vi "_CSMOFGV Dequeue.vi"(8 "Error in":errorcluster caption="Error in (no error)", 9 "Dequeue Timeout(0ms)":i32, 10 "State(s) in (\"\")":string, 11 "CSMQ in":T1={"Requested Name"="", "Module Name"="", "Mode"=enum."Stand Alone", "Queue"=refnum, "CSM-Data"=refnum, "User Event"=refnum, "Status Change Event"=refnum, "Allowed Messages"=[], "Mode-Data"=refnum, "Group Name"="", "Exit Event"=refnum}) -> (0 "Error out":errorcluster, 2 "States Out":string, 3 "CSMQ out":T1={"Requested Name"="", "Module Name"="", "Mode"=enum."Stand Alone", "Queue"=refnum, "CSM-Data"=refnum, "User Event"=refnum, "Status Change Event"=refnum, "Allowed Messages"=[], "Mode-Data"=refnum, "Group Name"="", "Exit Event"=refnum})   [LabVIEW 2020, in "Communicable State Machine.lvlib"]
uses:
  Communicable State Machine.lvlib
  _CSMObj.ctl
  Priority Queue.lvclass
  _CSM_MODE.ctl
  _CSMObj-Data.ctl
  _CSM Status Change Event Data.ctl
  _CSMObj-ModeData.ctl
  Priority Queue.lvclass/Priority Queue.ctl
  CSM - Convert Error to Argument.vi
  CSM - Make String Arguments Safe.vi
  CSM - Keywords.vi
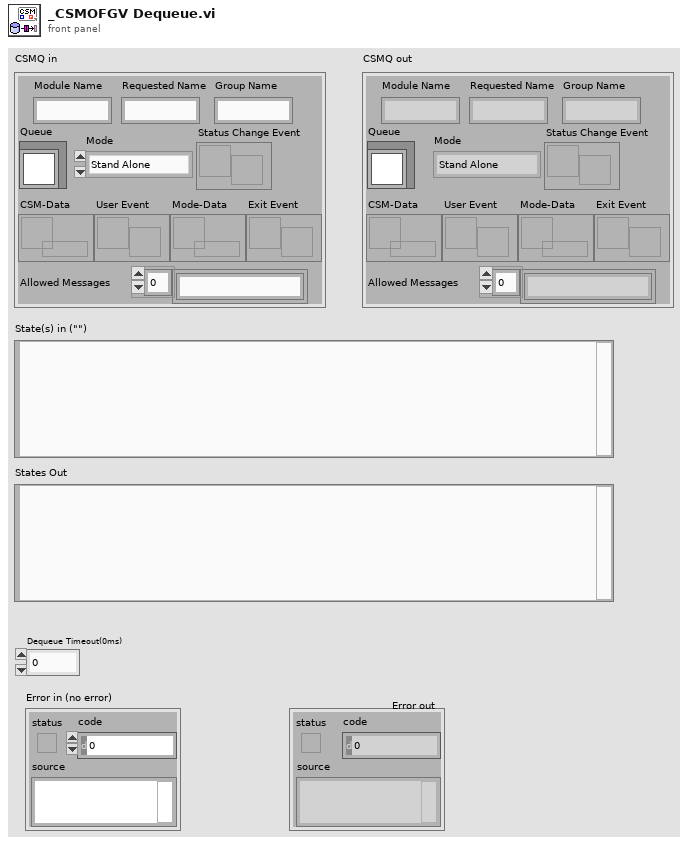
[diagram p1: front panel]
types:
  T1 = typedef "Communicable State Machine.lvlib/_CSMObj.ctl" = cluster{"Requested Name":string, "Module Name":string, "Mode":T2, "Queue":refnum<class "Priority Queue.lvclass">, "CSM-Data":refnum<data-value>, "User Event":refnum<user-event>, "Status Change Event":refnum<user-event>, "Allowed Messages":string[], "Mode-Data":refnum<data-value>, "Group Name":string, "Exit Event":refnum<user-event>}
  T2 = typedef "Communicable State Machine.lvlib/_CSM_MODE.ctl" = enum16{"Not Exist", "Stand Alone", "CSM", "Worker Agent", "Worker", "Chain", "Chain Node"}
  T3 = typedef "Communicable State Machine.lvlib/_CSMObj-Data.ctl" = cluster{"RemoteMessge?":bool, "error":errorcluster}
  T4 = typedef "Communicable State Machine.lvlib/_Cross CSM State Data.ctl" = cluster{"Msg Type":T5, "state":string, "args":string, "source":string, "RespQ":refnum<queue>, "Response For Message":T6, "Target":string}
  T5 = typedef "Communicable State Machine.lvlib/_CSM_MSG_TYPE.ctl" = enum16{"Sync Message(-@)", "Async Message(->)", "Async without Response(->|)", "Async Response", "Broadcast(-><all>)", "Broadcast(-><status>)", "Broadcast(-><interrupt>)", "Append to JKISM States", "Append to JKISM States(High Priority)"}
  T6 = typedef "Communicable State Machine.lvlib/_CSM_Response Source Message.ctl" = cluster{"‘State":string, "’Arguments":string, "’Error":errorcluster}
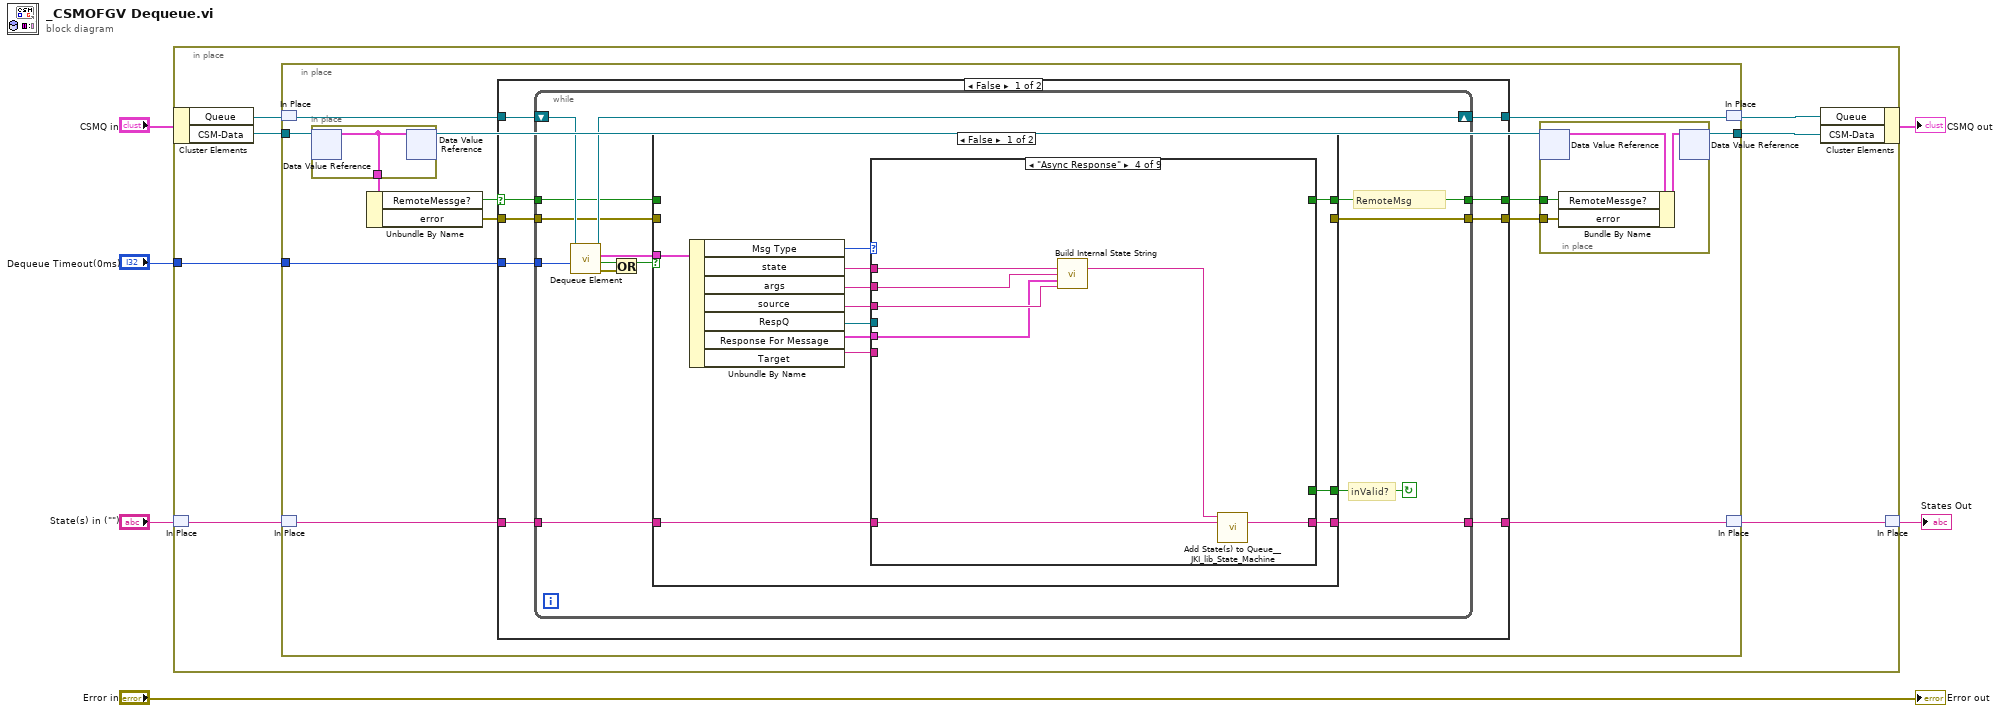
[diagram p0: block diagram]
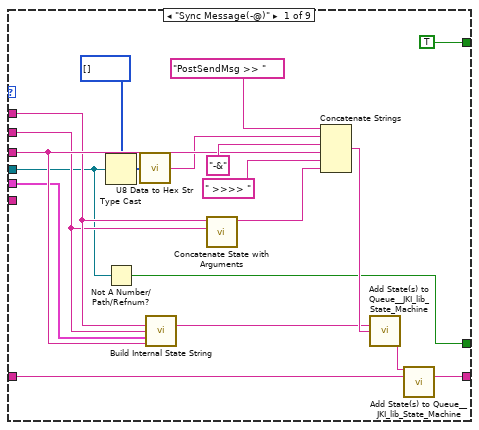
[diagram p2: hidden frame]
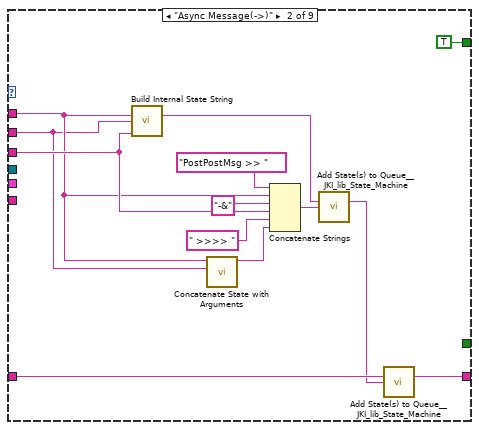
[diagram p3: hidden frame]
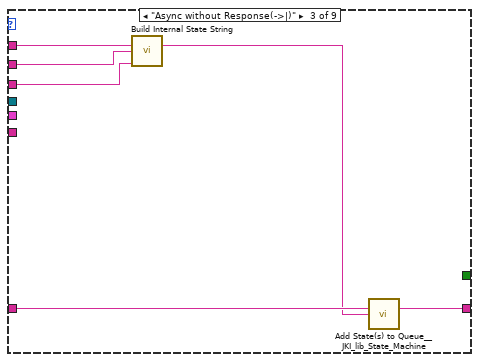
[diagram p4: hidden frame]
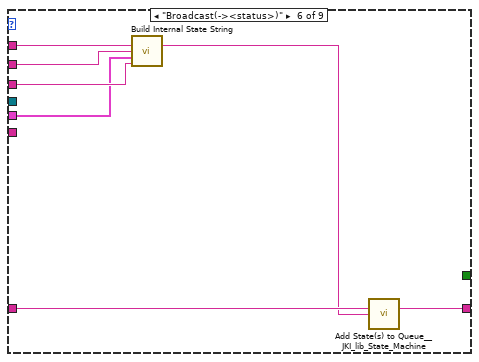
[diagram p6: hidden frame]
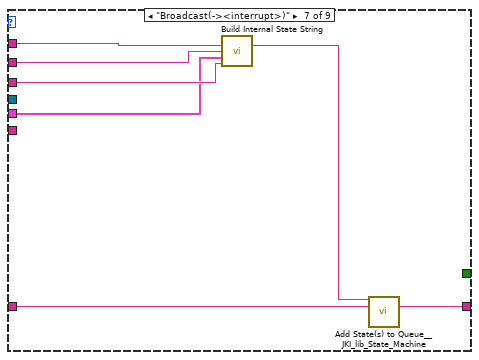
[diagram p7: hidden frame]
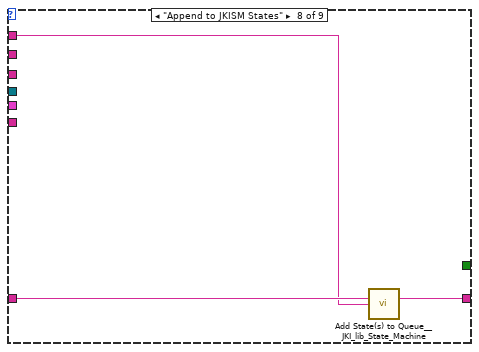
[diagram p8: hidden frame]
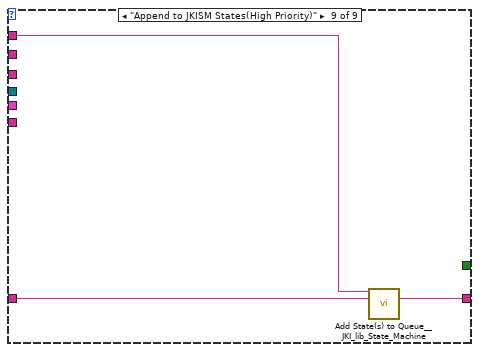
[diagram p9: hidden frame]
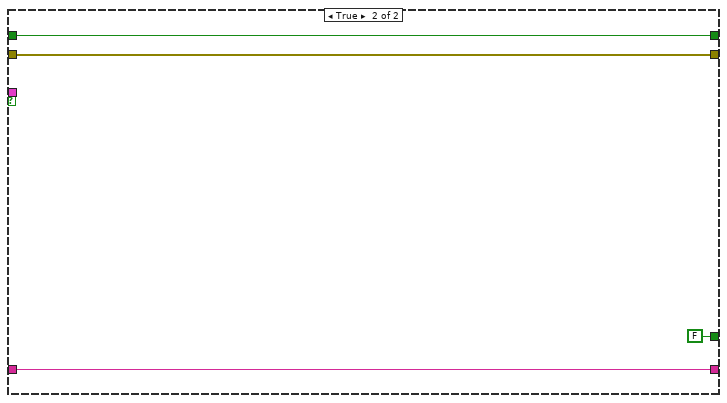
[diagram p10: hidden frame]
diagram:
  n1 = in-place "In Place Element Structure" {
    in-place-border: "Dequeue Timeout(0ms)" -> [w11]
    n2 = in-place-cluster #1("CSMQ in") -> ("Queue"=w13:refnum<class "Priority Queue.lvclass">, "CSM-Data"=w8:refnum<data-value>)
    n3 = in-place-match #2("State(s) in (\"\")") -> (w10:string)
    n4 = in-place {
      in-place-border: w11 -> [w24]
      in-place-border: w8 -> [w21]
      in-place-border: [w18] -> w7
      n5 = in-place-match #3(w13) -> (w25:refnum<class "Priority Queue.lvclass">)
      n6 = in-place-match #4(w10) -> (w23:string)
      n7 = in-place {
        in-place-border: [w31] -> w20
        n8 = in-place-dvr #5(w21) -> (w31:T3)  [unwired: 1 out]
        n9 = in-place-dvr #5(w31) -> (w19:refnum<data-value>)  [unwired: 1 out]
      }
      n10 = Unbundle By Name(w20) -> ("RemoteMessge?"=w16:bool, "error"=w14:errorcluster)
      n11 = case shown="False" w16 {
        selector: w16 -> [w34 w138]
        tunnel: [w39 w140] -> w26
        tunnel: w25 -> [w40 w140]
        tunnel: w24 -> [w38 _]
        tunnel: w23 -> [w37 w139]
        tunnel: [w36 w139] -> w22
        tunnel: [w35 w138] -> w17
        tunnel: [w33 w137] -> w15
        tunnel: w14 -> [w32 w137]
        frame False {
          n12 = while {
            tunnel: w38 -> [w52]
            shift-right: [w53] -> w39
            shift-left: w40 -> [w54]
            tunnel: w34 -> [w44]
            tunnel: [w45] -> w35
            tunnel: w37 -> [w50]
            tunnel: [w49] -> w36
            tunnel: [w42] -> w33
            tunnel: w32 -> [w41]
            stop <- w43 continue-if-true
            # "inValid?"
            # "RemoteMsg"
            n13 = call "Dequeue Element.vi"("timeout in ms (-1)"=w52, "Priority Queue"=w54) -> ("error out"=w46:errorcluster, "timed out?"=w47:bool, "Cross JKI State Machine State"=w51:T4, "Priority Queue(dup)"=w53:refnum<class "Priority Queue.lvclass">)  [unwired: 5 in, 1 out]
            n14 = Or(x=w47, y=w46) -> (x .or. y?=w48:bool)
            n15 = case shown="False" w48 {
              tunnel: w50 -> [w66 w136]
              tunnel: [w65 w136] -> w49
              tunnel: w51 -> [w60 _]
              tunnel: [w56 w135] -> w45
              tunnel: w44 -> [_ w135]
              tunnel: [w55 FALSE] -> w43
              tunnel: [_ w133] -> w42
              tunnel: w41 -> [_ w133]
              frame False {
                n16 = Unbundle By Name(w60) -> ("Msg Type"=w58:T5, "state"=w63:string, "args"=w62:string, "source"=w61:string, "RespQ"=w64:refnum<queue>, "Response For Message"=w59:T6, "Target"=w57:string)
                n17 = case shown="\"Async Response\"" w58 {
                  tunnel: w66 -> [w85 w98 w104 w111 w112 w119 w126 w129 w132]
                  tunnel: [w84 w97 w103 w110 w112 w118 w125 w128 w131] -> w65
                  tunnel: w64 -> [w68 _ _ _ _ _ _ _ _]
                  tunnel: w63 -> [w74 w87 w100 w107 _ w115 w122 w127 w130]
                  tunnel: w62 -> [w73 w86 w102 w109 _ w117 w124 _ _]
                  tunnel: w61 -> [w77 w96 w101 w108 _ w116 w123 _ _]
                  tunnel: w59 -> [w75 _ _ w105 _ w114 w121 _ _]
                  tunnel: w57 -> [_ _ _ _ _ _ _ _ _]
                  tunnel: [TRUE TRUE _ _ _ _ _ _ _] -> w56
                  tunnel: [w67 _ _ _ _ _ _ _ _] -> w55
                  frame "Sync Message(-@)" {
                    n18 = Type Cast(type=u8[] [], x=w68) -> (*(type *) &x=w70:u8[])
                    n19 = Not A Number/Path/Refnum?(number/path/refnum=w68) -> (NaN/Path/Refnum?=w67:bool)
                    n20 = call "U8 Data to Hex Str.vi"("u8 Data[]"=w70) -> ("HEX String (0-9,A-F)"=w69:string)
                    n21 = call "Build Internal State String.vi"("State"=w74, "Arguments (\"\")"=w73, ">> Response Source Message >>"=w75, "Source (\"\")"=w77) -> ("State with Arguments"=w80:string)  [unwired: 11 in]
                    n22 = call "Concatenate State with Arguments.vi"("Arguments"=w73, "State"=w74) -> ("State with Arguements"=w72:string)  [unwired: 9 in]
                    n23 = Concatenate Strings("PostSendMsg >> " ("State(s) at Back (\"\")"), w69, "-&" ("string"), w77, " >>>> " ("string"), w72) -> (w81:string)
                    n24 = call "Add State(s) to Queue__JKI_lib_State_Machine.vi"("State(s) in (\"\")"=w80, "State(s) at Back (\"\")"=w81) -> ("States Out"=w83:string)  [unwired: 13 in]
                    n25 = call "Add State(s) to Queue__JKI_lib_State_Machine.vi"("State(s) in Front (\"\")"=w83, "State(s) in (\"\")"=w85) -> ("States Out"=w84:string)  [unwired: 13 in]
                  }
                  frame "Async Message(->)" {
                    n26 = call "Build Internal State String.vi"("State"=w87, "Arguments (\"\")"=w86, "Source (\"\")"=w96) -> ("State with Arguments"=w92:string)  [unwired: 12 in]
                    n27 = call "Concatenate State with Arguments.vi"("Arguments"=w86, "State"=w87) -> ("State with Arguements"=w88:string)  [unwired: 9 in]
                    n28 = Concatenate Strings("PostPostMsg >> " ("State(s) at Back (\"\")"), w87, "-&" ("string"), w96, " >>>> " ("string"), w88) -> (w91:string)
                    n29 = call "Add State(s) to Queue__JKI_lib_State_Machine.vi"("State(s) in (\"\")"=w92, "State(s) at Back (\"\")"=w91) -> ("States Out"=w95:string)  [unwired: 13 in]
                    n30 = call "Add State(s) to Queue__JKI_lib_State_Machine.vi"("State(s) in (\"\")"=w98, "State(s) at Back (\"\")"=w95) -> ("States Out"=w97:string)  [unwired: 13 in]
                  }
                  frame "Async without Response(->|)" {
                    n31 = call "Build Internal State String.vi"("State"=w100, "Arguments (\"\")"=w102, "Source (\"\")"=w101) -> ("State with Arguments"=w99:string)  [unwired: 12 in]
                    n32 = call "Add State(s) to Queue__JKI_lib_State_Machine.vi"("State(s) in (\"\")"=w104, "State(s) at Back (\"\")"=w99) -> ("States Out"=w103:string)  [unwired: 13 in]
                  }
                  frame "Async Response" {
                    n33 = call "Build Internal State String.vi"("State"=w107, "Arguments (\"\")"=w109, ">> Response Source Message >>"=w105, "Source (\"\")"=w108) -> ("State with Arguments"=w106:string)  [unwired: 11 in]
                    n34 = call "Add State(s) to Queue__JKI_lib_State_Machine.vi"("State(s) in Front (\"\")"=w106, "State(s) in (\"\")"=w111) -> ("States Out"=w110:string)  [unwired: 13 in]
                  }
                  frame "Broadcast(-><all>)" {
                    # "#NOTE\nshould no be here"
                  }
                  frame "Broadcast(-><status>)" {
                    n35 = call "Build Internal State String.vi"("State"=w115, "Arguments (\"\")"=w117, ">> Response Source Message >>"=w114, "Source (\"\")"=w116) -> ("State with Arguments"=w113:string)  [unwired: 11 in]
                    n36 = call "Add State(s) to Queue__JKI_lib_State_Machine.vi"("State(s) in (\"\")"=w119, "State(s) at Back (\"\")"=w113) -> ("States Out"=w118:string)  [unwired: 13 in]
                  }
                  frame "Broadcast(-><interrupt>)" {
                    n37 = call "Build Internal State String.vi"("State"=w122, "Arguments (\"\")"=w124, ">> Response Source Message >>"=w121, "Source (\"\")"=w123) -> ("State with Arguments"=w120:string)  [unwired: 11 in]
                    n38 = call "Add State(s) to Queue__JKI_lib_State_Machine.vi"("State(s) in Front (\"\")"=w120, "State(s) in (\"\")"=w126) -> ("States Out"=w125:string)  [unwired: 13 in]
                  }
                  frame "Append to JKISM States" {
                    n39 = call "Add State(s) to Queue__JKI_lib_State_Machine.vi"("State(s) in (\"\")"=w129, "State(s) at Back (\"\")"=w127) -> ("States Out"=w128:string)  [unwired: 13 in]
                  }
                  frame "Append to JKISM States(High Priority)" {
                    n40 = call "Add State(s) to Queue__JKI_lib_State_Machine.vi"("State(s) in Front (\"\")"=w130, "State(s) in (\"\")"=w132) -> ("States Out"=w131:string)  [unwired: 13 in]
                  }
                }
              }
              frame True {
              }
            }
          }
        }
        frame True {
        }
      }
      n41 = in-place {
        in-place-border: w17 -> [w28]
        in-place-border: w15 -> [w27]
        n42 = in-place-dvr #6(w19) -> (w30:T3)  [unwired: 1 out]
        n43 = Bundle By Name(cluster=w30, "RemoteMessge?"=w28, "error"=w27) -> (w29:T3)
        n44 = in-place-dvr #6(w29) -> (w18:refnum<data-value>)  [unwired: 1 out]
      }
      n45 = in-place-match #3(w26) -> (w12:refnum<class "Priority Queue.lvclass">)
      n46 = in-place-match #4(w22) -> (w9:string)
    }
    n47 = in-place-cluster #1("Queue"=w12, "CSM-Data"=w7) -> (→"CSMQ out":T1)
    n48 = in-place-match #2(w9) -> (→"States Out":string)
  }
  "Error out" <- "Error in"
